vi "Main_EEG_Feature_Extraction.vi"() -> ()   [LabVIEW 2023]
panel:
  in  "File Path":path
  in  "Lower Cut-Off\nfor Lowpass Filter":dbl=70.0
  in  "Higher Cut-Off\nfor Highpass Filter":dbl=1.0
  in  "Upper Cut-Off\nfor Notch Filter":dbl=60.0 caption="Upper Cut-Off"
  in  "Lower Cut-Off\nfor Notch Filter":dbl=45.0 caption="Lower Cut-Off"
  in  "Sampling Frequency\nfor  Bandpass Filtering":dbl=512.0
  in  "Absolute\nData":bool
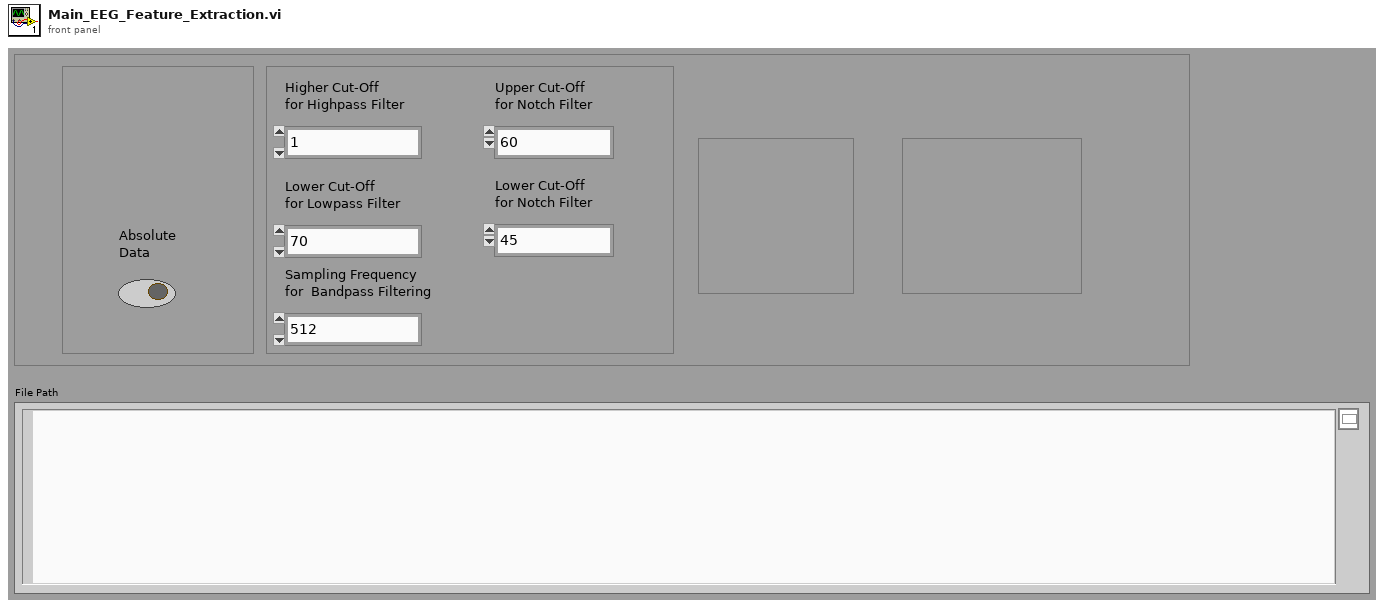
[diagram p1: front panel]
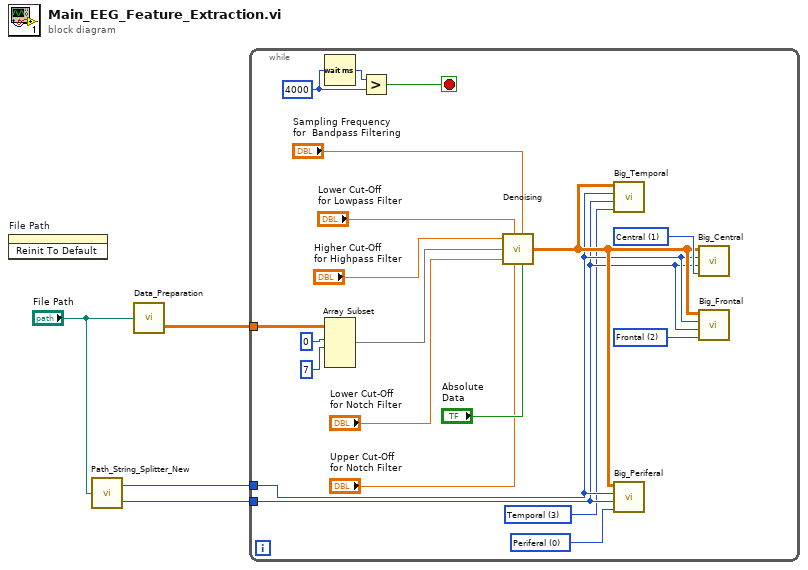
[diagram p0: block diagram]
diagram:
  n1 = invoke on="File Path" class="Path" method="Reinit To Default"() -> ()  [unwired: 3 in, 3 out]
  n2 = call "Path_String_Splitter_New.vi"("File Path"="File Path") -> ("Experment Index"=w2:i32, "Session Index"=w1:i32)
  n3 = call "Data_Preparation.vi"("File Path"="File Path") -> ("Datas"=w4:dbl[][])  [unwired: 1 out]
  n4 = while {
    tunnel: w4 -> [w24]
    tunnel: w2 -> [w10]
    tunnel: w1 -> [w9]
    stop <- w5 stop-if-true
    w12 = u16 2 items=["Periferal", "Central", "Frontal", "Temporal"] ("Feature Selection Output")
    w8 = u16 3 items=["Periferal", "Central", "Frontal", "Temporal"] ("Feature Selection Output")
    w14 = u16 0 items=["Periferal", "Central", "Frontal", "Temporal"] ("Feature Selection Output")
    w13 = u16 1 items=["Periferal", "Central", "Frontal", "Temporal"] ("Feature Selection Output")
    w6 = u32 4000 ("milliseconds to wait")
    n5 = Wait (ms)(milliseconds to wait=w6) -> (millisecond timer value=w7:u32)
    n6 = Array Subset "Array Subset"(array=w24, index (row)=0 ("index"), length (row)=7 ("length")) -> (w20:dbl[][])  [unwired: 2 in]
    n7 = Greater?(x=w7, y=w6) -> (0:w5:bool)
    n8 = call "Denoising.vi"("Higher Cut-Off\nfor Highpass Filter"="Higher Cut-Off\nfor Highpass Filter", "Lower Cut-Off\nfor Lowpass Filter"="Lower Cut-Off\nfor Lowpass Filter", "Array in"=w20, "Lower Cut-Off\nfor Notch Filter"="Lower Cut-Off\nfor Notch Filter", "Upper Cut-Off\nfor Notch Filter"="Upper Cut-Off\nfor Notch Filter", "Sampling Frequency\nfor  Bandpass Filtering"="Sampling Frequency\nfor  Bandpass Filtering", "Absolute Data"="Absolute\nData") -> ("Array out"=w11:dbl[][])  [unwired: 2 in]
    n9 = call "Big_Temporal.vi"("Feature Selection"=w8, "Session Index"=w9, "Experment Index"=w10, "Array in"=w11) -> ()  [unwired: 3 out]
    n10 = call "Big_Periferal.vi"("Feature Selection"=w14, "Session Index"=w9, "Experment Index"=w10, "Array in"=w11) -> ()  [unwired: 3 out]
    n11 = call "Big_Central.vi"("Feature Selection"=w13, "Session Index"=w9, "Experment Index"=w10, "Array in"=w11) -> ()  [unwired: 3 out]
    n12 = call "Big_Frontal.vi"("Feature Selection"=w12, "Session Index"=w9, "Experment Index"=w10, "Array in"=w11) -> ()  [unwired: 3 out]
  }
